vi "XWPF Writer - Add Picture Tests.vi"(8 "error in (no error)":errorcluster) -> (0 "error out":errorcluster)   [LabVIEW 2017]
uses:
  <vilib>/addons/_JKI Toolkits/Caraya/classes/Assert/Assert Not Error.vi
  <vilib>/addons/_JKI Toolkits/Caraya/classes/Assert/Assert True.vi
  src/LabVIEW NPOI/xwpfWriter/xwpfWriter.lvclass
  <vilib>/addons/_JKI Toolkits/Caraya/classes/Test/Test.lvclass
  <vilib>/addons/_JKI Toolkits/Caraya/classes/Assert/Assert.lvclass
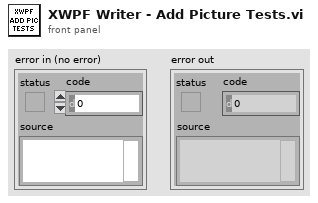
[diagram p1: front panel]
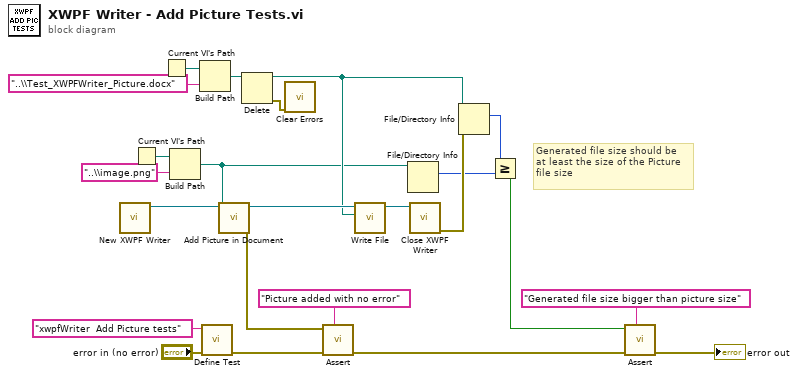
[diagram p0: block diagram]
diagram:
  # "Generated file size should be\nat least the size of the Picture \nfile size"
  n1 = call "New XWPF Writer.vi"() -> ("xwpfWriter out"=w15:refnum<class "xwpfWriter.lvclass">)  [unwired: 10 in, 1 out]
  n2 = Current VI's Path() -> (path=w10:path)
  n3 = Current VI's Path() -> (path=w13:path)
  n4 = Build Path(base path=w10, name or relative path="..\\image.png" ("string")) -> (appended path=w4:path)
  n5 = Build Path(base path=w13, name or relative path="..\\Test_XWPFWriter_Picture.docx" ("string")) -> (appended path=w12:path)
  n6 = call <vilib>:"Define Test.vi"("error in (no error)"="error in (no error)", "Label (VI Title)"="xwpfWriter  Add Picture tests") -> ("error out"=w19:errorcluster)  [unwired: 9 in]
  n7 = call "Add Picture in Document.vi"("Picture Path"=w4, "xwpfWriter in"=w15) -> ("error out"=w8:errorcluster, "xwpfWriter out"=w22:refnum<class "xwpfWriter.lvclass">)  [unwired: 8 in]
  n8 = Delete(path (use dialog)=w12) -> (deleted path=w7:path, error out=w11:errorcluster)  [unwired: 4 in, 1 out]
  n9 = call <vilib>:"Clear Errors.vi"("error in (no error)"=w11) -> ()  [unwired: 5 in, 2 out]
  n10 = call-poly <vilib>:"Assert.vi"("Label"="Picture added with no error", "error in (no error)"=w19, "Not Error?"=w8) -> ("error out"=w16:errorcluster)  [unwired: 8 in]
  n11 = call "Write File.vi"("path"=w7, "xwpfWriter in"=w22) -> ("xwpfWriter out"=w23:refnum<class "xwpfWriter.lvclass">)  [unwired: 8 in, 1 out]
  n12 = File/Directory Info(path=w4) -> (size=w2:i64)  [unwired: 1 in, 6 out]
  n13 = call "Close XWPF Writer.vi"("xwpfWriter in"=w23) -> ("error out"=w6:errorcluster)  [unwired: 9 in, 1 out]
  n14 = File/Directory Info(path=w7, error in=w6) -> (size=w3:i64)  [unwired: 6 out]
  n15 = Greater Or Equal?(x=w3, y=w2) -> (x >= y?=w1:bool)
  n16 = call-poly <vilib>:"Assert.vi"("Label"="Generated file size bigger than picture size", "error in (no error)"=w16, "True?"=w1) -> ("error out"=→"error out":errorcluster)  [unwired: 8 in]
